vi "clustertest.vi"() -> ()   [LabVIEW 2010]
panel:
  out "Bauteil1":i32[][](array[numeric])
  out "Bauteil0":i32[][](array[numeric])
  in  "Methode":i32
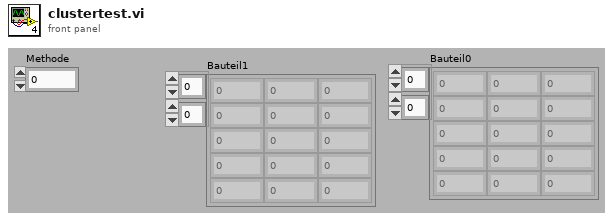
[diagram p1: front panel]
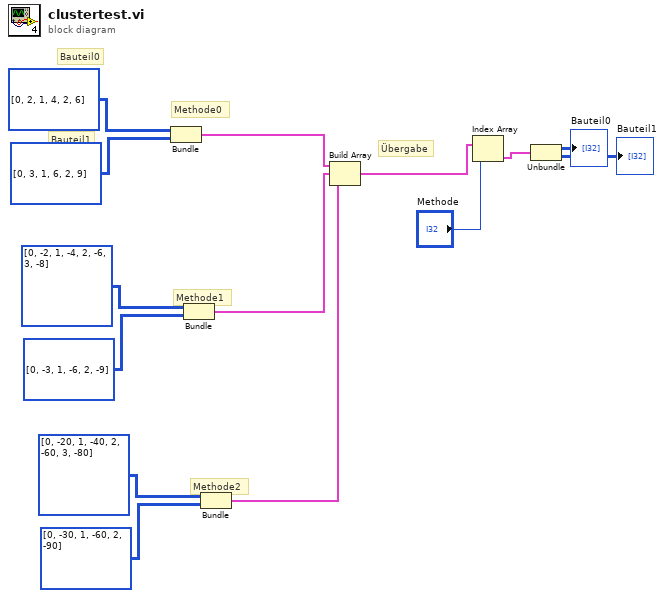
[diagram p0: block diagram]
diagram:
  # "Methode2"
  # "Übergabe"
  # "Bauteil1"
  # "Bauteil0"
  # "Methode1"
  # "Methode0"
  n1 = Bundle(i32[][] [[0, 2], [1, 4], [2, 6]], i32[][] [[0, 3], [1, 6], [2, 9]]) -> (w10:cluster{i32[][], i32[][]})  [unwired: 1 in]
  n2 = Bundle(i32[][] [[0, -2], [1, -4], [2, -6], [3, -8]], i32[][] [[0, -3], [1, -6], [2, -9]]) -> (w9:cluster{i32[][], i32[][]})  [unwired: 1 in]
  n3 = Bundle(i32[][] [[0, -20], [1, -40], [2, -60], [3, -80]], i32[][] [[0, -30], [1, -60], [2, -90]]) -> (w1:cluster{i32[][], i32[][]})  [unwired: 1 in]
  n4 = Build Array(w10, w9, w1) -> (w8:cluster{i32[][], i32[][]}[])
  n5 = Index Array(array=w8, index="Methode") -> (element=w6:cluster{i32[][], i32[][]})
  n6 = Unbundle(w6) -> (→"Bauteil0":i32[][], →"Bauteil1":i32[][])
